vi "FlatToRichrfcontrol_GetGPSLastLocInfoRequest.vi"(5 "OutputClusterType":T1, 11 "InputCluster":T2) -> (3 "OutputCluster":T1)   [LabVIEW 2024, in "FlexSDR_gRPC_client.lvlib"]
uses:
  rfcontrol_GetGPSLastLocInfoRequest_Flat.ctl
  rfcontrol_GetGPSLastLocInfoRequest.ctl
  FlexSDR_gRPC_client.lvlib
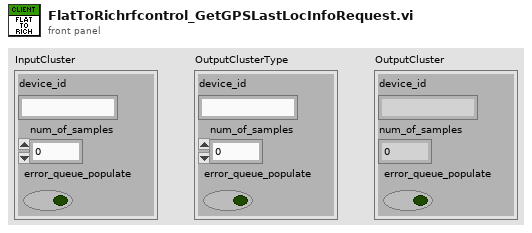
[diagram p1: front panel]
types:
  T1 = typedef "FlexSDR_gRPC_client.lvlib/rfcontrol_GetGPSLastLocInfoRequest.ctl" = cluster{"device_id":string, "num_of_samples":i32, "error_queue_populate":bool}
  T2 = typedef "FlexSDR_gRPC_client.lvlib/rfcontrol_GetGPSLastLocInfoRequest_Flat.ctl" = cluster{"device_id":string, "num_of_samples":i32, "error_queue_populate":bool}
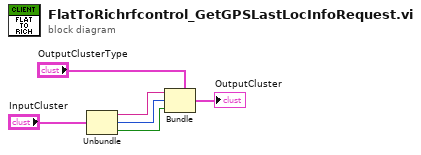
[diagram p0: block diagram]
diagram:
  n1 = Unbundle "Unbundle"("InputCluster") -> ("device_id"=w3:string, "num_of_samples"=w2:i32, "error_queue_populate"=w1:bool)
  n2 = Bundle "Bundle"(cluster="OutputClusterType", "device_id"=w3, "num_of_samples"=w2, "error_queue_populate"=w1) -> (→"OutputCluster":T1)
